vi "Remakecase.vi"   [LabVIEW 2015]
uses:
  <vilib>/NXT/Block Support/NXT_InputPort.ctl
  <vilib>/NXT/Block Support/NXT_OutputPort.ctl
  <vilib>/NXT/Dual Mode Library/Sensors/Light_On.vi
  <vilib>/NXT/Dual Mode Library/Sensors/Sonar_cm.vi
  <vilib>/NXT/NXTIO Xnodes/NXTIONodeSubVIs/NXTMoveMotors.vi
  <vilib>/NXT/Dual Mode Library/Waits/Wait_Num(msec).vi
  <vilib>/NXT/Subs/LVHSConnector.ctl
  <vilib>/NXT/NXTIO Xnodes/AddressXNode/NXTIOAddress.xnode
  <vilib>/NXT/NXTIO Xnodes/NXTIOXNode/NXTIO.xnode
  <vilib>/NXT/LegoClasses/BrickReference/BrickReference.lvclass
types:
  T1 = typedef "NXT_OutputPort.ctl" = u8
  T2 = typedef "NXT_InputPort.ctl" = u32
  T3 = typedef "LVHSConnector.ctl" = refnum<class "BrickReference.lvclass">
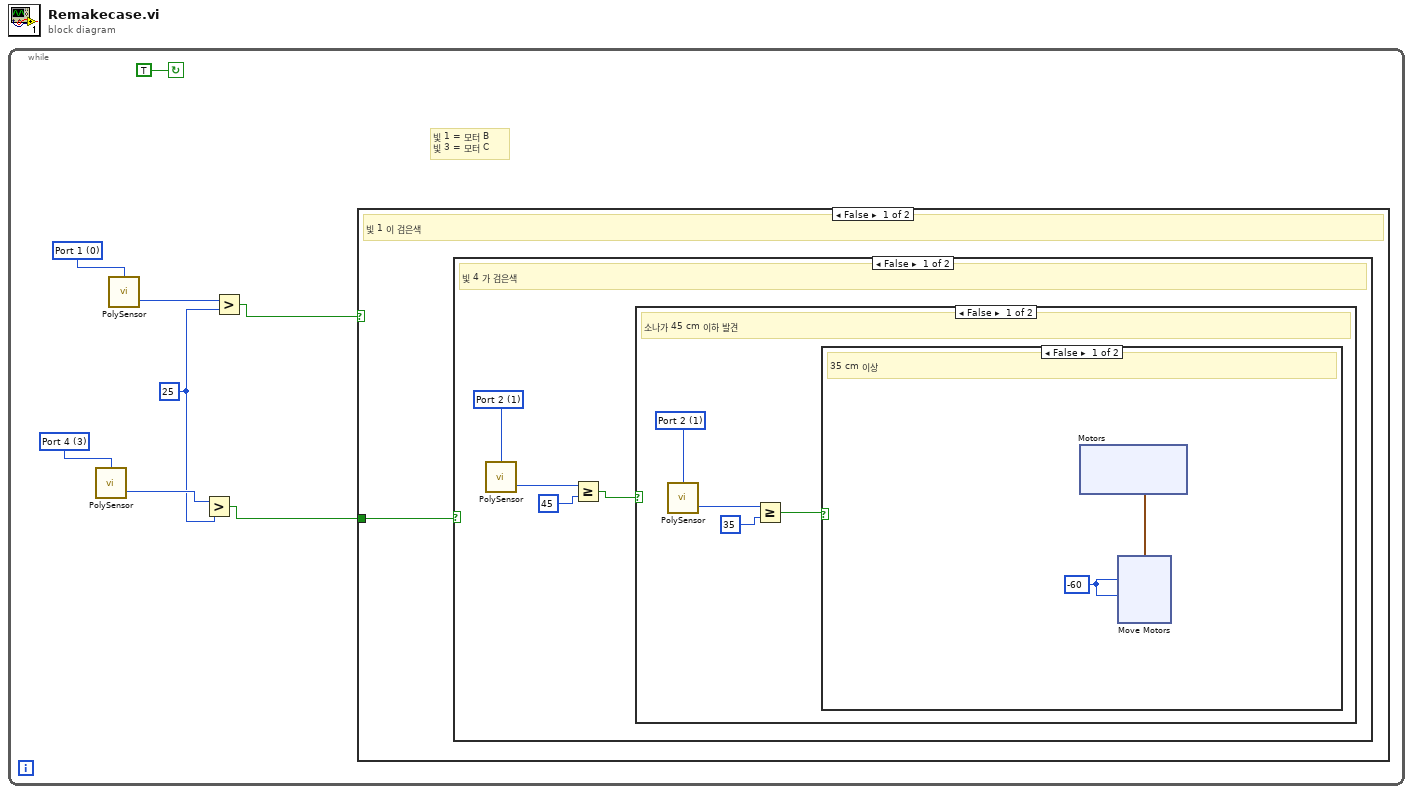
[diagram p0: block diagram]
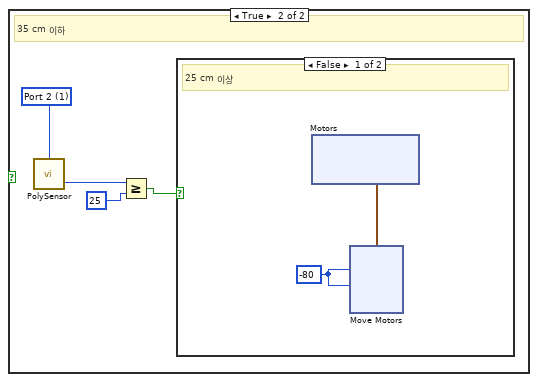
[diagram p2: hidden frame]
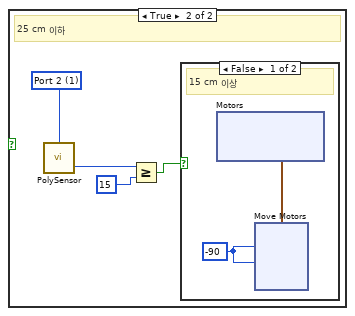
[diagram p3: hidden frame]
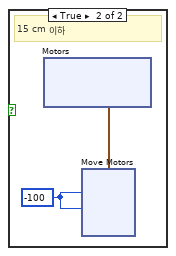
[diagram p4: hidden frame]
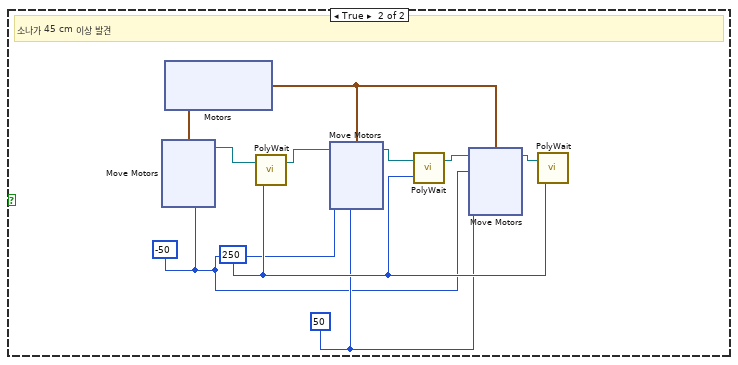
[diagram p5: hidden frame]
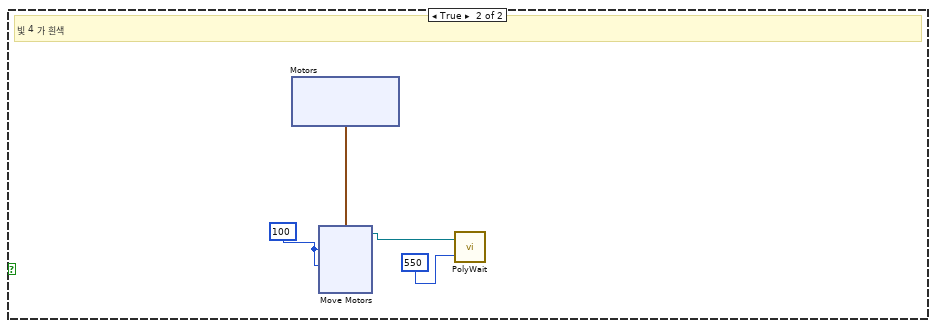
[diagram p6: hidden frame]
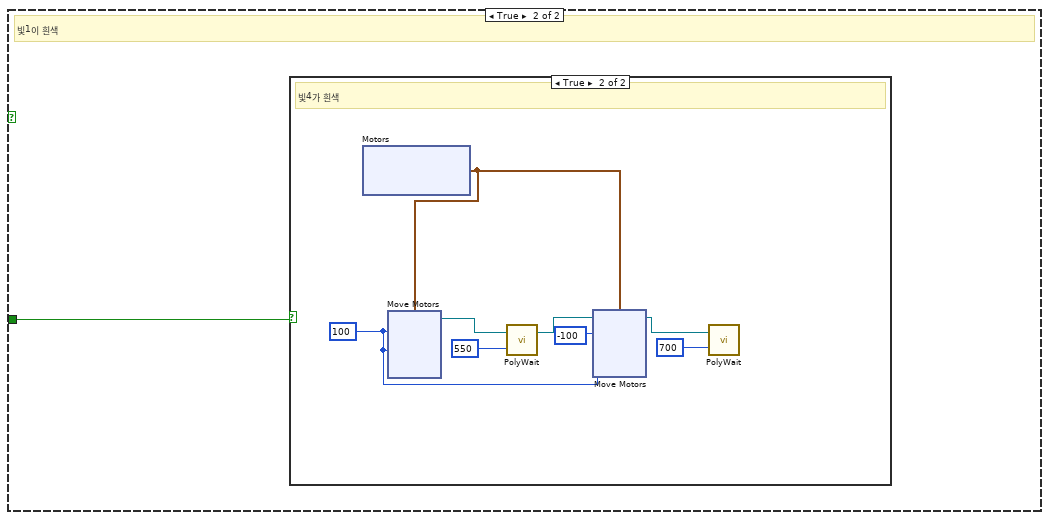
[diagram p7: hidden frame]
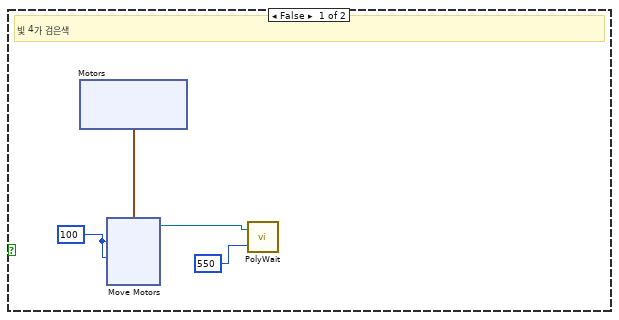
[diagram p8: hidden frame]
diagram:
  n1 = while {
    stop <- TRUE continue-if-true
    w1 = i16 25 ("y")
    w6 = T2 0 items=["Port 1", "Port 2", "Port 3", "Port 4"] ("Port (Port 3)")
    w5 = T2 3 items=["Port 1", "Port 2", "Port 3", "Port 4"] ("Port (Port 3)")
    # "빛 1 = 모터 B\n빛 3 = 모터 C"
    n2 = call-poly <vilib>:"PolySensor.vi"("Port (Port 3)"=w5) -> ("Scaled Value"=w7:i16)  [unwired: 2 in, 1 out]
    n3 = call-poly <vilib>:"PolySensor.vi"("Port (Port 3)"=w6) -> ("Scaled Value"=w8:i16)  [unwired: 2 in, 1 out]
    n4 = Greater?(x=w7, y=w1) -> (0:w3:bool)
    n5 = Greater?(x=w8, y=w1) -> (0:w4:bool)
    n6 = case shown="False" w4 {
      tunnel: w3 -> [w9 w117]
      frame False {
        # "빛 1 이 검은색"
        n7 = case shown="False" w9 {
          frame False {
            w10 = T2 1 items=["Port 1", "Port 2", "Port 3", "Port 4"] ("Port (Port 4)")
            # "빛 4 가 검은색"
            n8 = call-poly <vilib>:"PolySensor.vi"("Port (Port 4)"=w10) -> ("Distance (cm)"=w13:i16)  [unwired: 2 in, 1 out]
            n9 = Greater Or Equal?(x=w13, y=i16 45) -> (x >= y?=w11:bool)
            n10 = case shown="False" w11 {
              frame False {
                w15 = T2 1 items=["Port 1", "Port 2", "Port 3", "Port 4"] ("Port (Port 4)")
                # "소나가 45 cm 이하 발견"
                n11 = call-poly <vilib>:"PolySensor.vi"("Port (Port 4)"=w15) -> ("Distance (cm)"=w17:i16)  [unwired: 2 in, 1 out]
                n12 = Greater Or Equal?(x=w17, y=i16 35) -> (x >= y?=w14:bool)
                n13 = case shown="False" w14 {
                  frame False {
                    w18 = i16 -60 ("y")
                    # "35 cm 이상"
                    n14 = xnode "Motors"() -> ("Motor"=w19:cluster{"Port":T1, "Port":T1})
                    n15 = xnode "Move Motors"("Power/Speed 2"=w18, "Power/Speed 1"=w18, "Motors"=w19) -> ()  [unwired: 1 in, 1 out]
                  }
                  frame True {
                    w30 = T2 1 items=["Port 1", "Port 2", "Port 3", "Port 4"] ("Port (Port 4)")
                    # "35 cm 이하"
                    n16 = call-poly <vilib>:"PolySensor.vi"("Port (Port 4)"=w30) -> ("Distance (cm)"=w32:i16)  [unwired: 2 in, 1 out]
                    n17 = Greater Or Equal?(x=w32, y=i16 25) -> (x >= y?=w29:bool)
                    n18 = case shown="False" w29 {
                      frame False {
                        w33 = i16 -80 ("y")
                        # "25 cm 이상"
                        n19 = xnode "Motors"() -> ("Motor"=w34:cluster{"Port":T1, "Port":T1})
                        n20 = xnode "Move Motors"("Power/Speed 2"=w33, "Power/Speed 1"=w33, "Motors"=w34) -> ()  [unwired: 1 in, 1 out]
                      }
                      frame True {
                        w45 = T2 1 items=["Port 1", "Port 2", "Port 3", "Port 4"] ("Port (Port 4)")
                        # "25 cm 이하"
                        n21 = call-poly <vilib>:"PolySensor.vi"("Port (Port 4)"=w45) -> ("Distance (cm)"=w47:i16)  [unwired: 2 in, 1 out]
                        n22 = Greater Or Equal?(x=w47, y=i16 15) -> (x >= y?=w44:bool)
                        n23 = case shown="False" w44 {
                          frame False {
                            w48 = i16 -90 ("y")
                            # "15 cm 이상"
                            n24 = xnode "Motors"() -> ("Motor"=w49:cluster{"Port":T1, "Port":T1})
                            n25 = xnode "Move Motors"("Power/Speed 2"=w48, "Power/Speed 1"=w48, "Motors"=w49) -> ()  [unwired: 1 in, 1 out]
                          }
                          frame True {
                            w59 = i16 -100 ("y")
                            # "15 cm 이하"
                            n26 = xnode "Motors"() -> ("Motor"=w60:cluster{"Port":T1, "Port":T1})
                            n27 = xnode "Move Motors"("Power/Speed 2"=w59, "Power/Speed 1"=w59, "Motors"=w60) -> ()  [unwired: 1 in, 1 out]
                          }
                        }
                      }
                    }
                  }
                }
              }
              frame True {
                w77 = i16 250 ("y")
                w76 = i16 50 ("y")
                w75 = i16 -50 ("y")
                # "소나가 45 cm 이상 발견"
                n28 = xnode "Motors"() -> ("Motor"=w78:cluster{"Port":T1, "Port":T1})
                n29 = xnode "Move Motors"("Power/Speed 2"=w75, "Power/Speed 1"=w75, "Motors"=w78) -> ("NXT/EV3"=w74:T3)  [unwired: 1 in]
                n30 = call-poly <vilib>:"PolyWait.vi"("Time (100 msec)"=w77, "NXT/EV3"=w74) -> ("NXT/EV3"=w73:T3)  [unwired: 2 in]
                n31 = xnode "Move Motors"("Power/Speed 2"=w75, "Power/Speed 1"=w76, "Motors"=w78, "NXT/EV3"=w73) -> ("NXT/EV3"=w72:T3)
                n32 = call-poly <vilib>:"PolyWait.vi"("Time (100 msec)"=w77, "NXT/EV3"=w72) -> ("NXT/EV3"=w71:T3)  [unwired: 2 in]
                n33 = xnode "Move Motors"("Power/Speed 2"=w76, "Power/Speed 1"=w75, "Motors"=w78, "NXT/EV3"=w71) -> ("NXT/EV3"=w70:T3)
                n34 = call-poly <vilib>:"PolyWait.vi"("Time (100 msec)"=w77, "NXT/EV3"=w70) -> ()  [unwired: 2 in, 1 out]
              }
            }
          }
          frame True {
            w104 = i16 100 ("y")
            # "빛 4 가 흰색"
            n35 = xnode "Motors"() -> ("Motor"=w107:cluster{"Port":T1, "Port":T1})
            n36 = xnode "Move Motors"("Power/Speed 2"=w104, "Power/Speed 1"=w104, "Motors"=w107) -> ("NXT/EV3"=w105:T3)  [unwired: 1 in]
            n37 = call-poly <vilib>:"PolyWait.vi"("Time (100 msec)"=i16 550 ("y"), "NXT/EV3"=w105) -> ()  [unwired: 2 in, 1 out]
          }
        }
      }
      frame True {
        # "빛1이 흰색"
        n38 = case shown="True" w117 {
          frame False {
            w118 = i16 100 ("y")
            # "빛 4가 검은색"
            n39 = xnode "Motors"() -> ("Motor"=w121:cluster{"Port":T1, "Port":T1})
            n40 = xnode "Move Motors"("Power/Speed 2"=w118, "Power/Speed 1"=w118, "Motors"=w121) -> ("NXT/EV3"=w119:T3)  [unwired: 1 in]
            n41 = call-poly <vilib>:"PolyWait.vi"("Time (100 msec)"=i16 550 ("y"), "NXT/EV3"=w119) -> ()  [unwired: 2 in, 1 out]
          }
          frame True {
            w131 = i16 100 ("y")
            # "빛4가 흰색"
            n42 = xnode "Motors"() -> ("Motor"=w138:cluster{"Port":T1, "Port":T1})
            n43 = xnode "Move Motors"("Power/Speed 2"=w131, "Power/Speed 1"=w131, "Motors"=w138) -> ("NXT/EV3"=w137:T3)  [unwired: 1 in]
            n44 = call-poly <vilib>:"PolyWait.vi"("Time (100 msec)"=i16 550 ("y"), "NXT/EV3"=w137) -> ("NXT/EV3"=w136:T3)  [unwired: 2 in]
            n45 = xnode "Move Motors"("Power/Speed 2"=w131, "Power/Speed 1"=i16 -100 ("y"), "Motors"=w138, "NXT/EV3"=w136) -> ("NXT/EV3"=w135:T3)
            n46 = call-poly <vilib>:"PolyWait.vi"("Time (100 msec)"=i16 700 ("y"), "NXT/EV3"=w135) -> ()  [unwired: 2 in, 1 out]
          }
        }
      }
    }
  }
